vi "FeedForTime.vi"() -> ()   [LabVIEW 2020]
uses:
  Framework/Robot Global Data.vi
panel:
  in  "NoWait":bool
  in  "LowerSpeed":dbl
  in  "UpperSpeed":dbl
  in  "Time":dbl
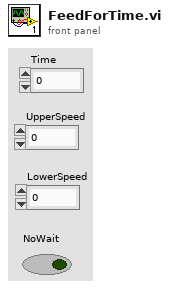
[diagram p1: front panel]
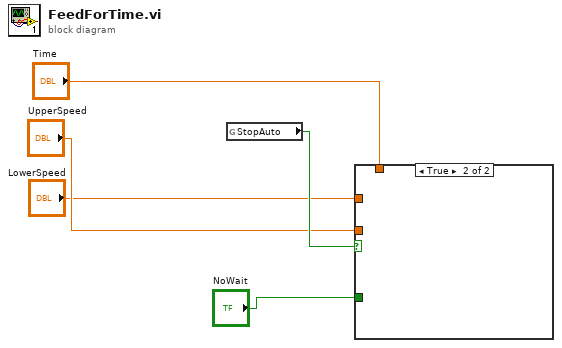
[diagram p0: block diagram]
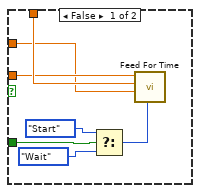
[diagram p2: hidden frame]
diagram:
  n1 = global read "Robot Global Data.vi" "StopAuto"() -> (w5:bool)
  n2 = case shown="True" w5 {
    tunnel: "NoWait" -> [w10 _]
    tunnel: "Time" -> [w8 _]
    tunnel: "UpperSpeed" -> [w7 _]
    tunnel: "LowerSpeed" -> [w6 _]
    frame False {
      n3 = Select(t=enum16{"Start", "Wait"}."Start" ("Synchronization"), s=w10, f=enum16{"Start", "Wait"}."Wait" ("Synchronization")) -> (s? t:f=w9:enum16{"Start", "Wait"})
      n4 = call "Feed For Time.vi"("Synchronization"=w9, "Lower"=w6, "Duration (s)"=w8, "Upper"=w7) -> ()  [unwired: 7 in, 1 out]
    }
    frame True {
    }
  }
